vi "setSettings.vi"(8 "error in (no error)":errorcluster, 11 "SEDSpectrometer in":refnum<class "SEDSpectrometer.lvclass">) -> (0 "error out":errorcluster, 3 "SEDSpectrometer out":refnum<class "SEDSpectrometer.lvclass">)   [LabVIEW 2016, in "SEDSpectrometer.lvclass"]
uses:
  SEDSpectrometer.lvclass
panel:
  in  "NrOfAVG":u32=1 caption="Number of averages"
  in  "IntDelay":dbl=-20.0 caption="Integration delay [ns]" min=-20.0 format="%#.0f"
  in  "IntTime":sgl=32.0 caption="Integration time [ms]" format="%.2f"
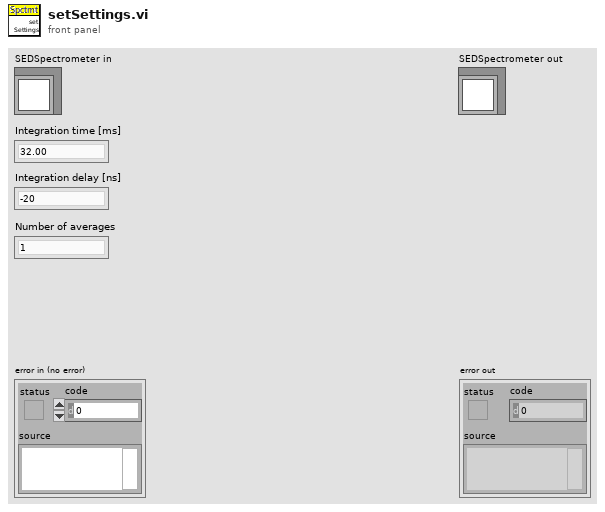
[diagram p1: front panel]
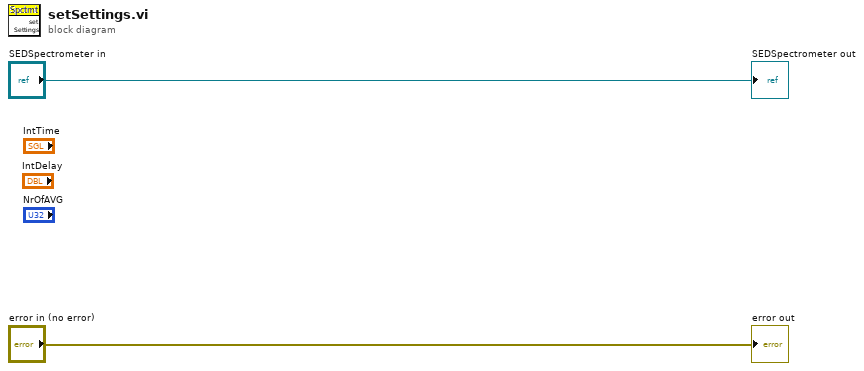
[diagram p0: block diagram]
diagram:
  "error out" <- "error in (no error)"
  "SEDSpectrometer out" <- "SEDSpectrometer in"
